vi "WalkOffSuite.vi"(6 "Stop on 1st fail":bool, 7 "Banana":refnum<class "Banana.lvclass">, 8 "error in (no error)":errorcluster, 11 "Leaf.TestSuite":refnum<class "Leaf.TestSuite.lvclass">) -> (0 "error out":errorcluster, 3 "Leaf.TestSuite":refnum<class "Leaf.TestSuite.lvclass">)   [LabVIEW 2021, in "Bananas.lvlib" / "Platano.lvclass"]
uses:
  Leaf.TestSuite/Leaf.TestSuite.lvclass
  Banana/Banana.lvclass
  Banana/Banana.lvclass/Banana.ctl
  BananaPeel/BananaPeel.lvclass
  Platano.lvclass
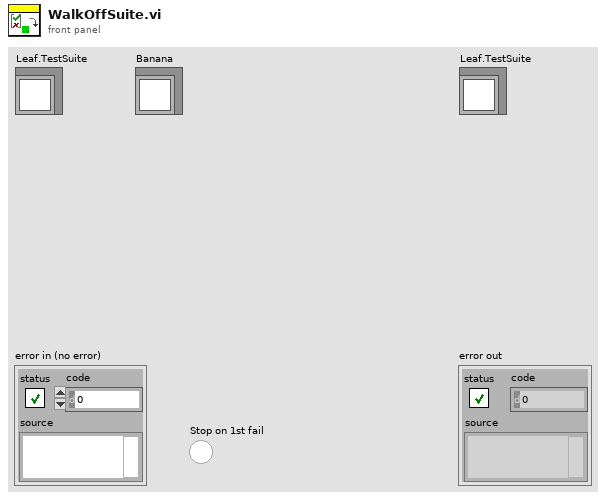
[diagram p1: front panel]
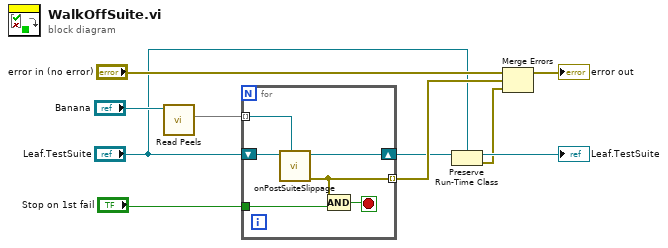
[diagram p0: block diagram]
diagram:
  n1 = call "Read Peels.vi"("Banana in"="Banana") -> ("Peels"=w5:set{refnum<class "BananaPeel.lvclass">})  [unwired: 8 in, 2 out]
  n2 = for {
    tunnel: [w11] -> w10 mode=indexing
    shift-right: [w12] -> w3
    shift-left: "Leaf.TestSuite" -> [w14]
    tunnel: w5 -> [w13] mode=indexing
    tunnel: "Stop on 1st fail" -> [w16]
    stop <- w15 stop-if-true
    n3 = call-dynamic "onPostSuiteSlippage.vi"("BananaPeel in"=w13, "Leaf.TestSuite"=w14) -> ("error out"=w11:errorcluster, "Leaf.TestSuite"=w12:refnum<class "Leaf.TestSuite.lvclass">)  [unwired: 8 in]
    n4 = Compound Arithmetic op=AND(w11, w16) -> (w15:bool)
  }
  n5 = Preserve Run-Time Class(object in=w3, 2:"Leaf.TestSuite") -> (object out=→"Leaf.TestSuite":refnum<class "Leaf.TestSuite.lvclass">, error out=w1:errorcluster)  [unwired: 1 in]
  n6 = Merge Errors("error in (no error)", w10, w1) -> (→"error out":errorcluster)
